vi "读取生成ncx.vi"(8 "error in (no error)":errorcluster caption="错误输入（无错误）", 11 "EPUB输入":refnum<class "EPUB.lvclass">) -> (0 "error out":errorcluster caption="错误输出", 2 "toc.ncx":string, 3 "EPUB输出":refnum<class "EPUB.lvclass">)   [LabVIEW 2016, in "EPUB.lvclass"]
uses:
  EPUB.lvclass
  EPUB.lvclass/EPUB.ctl
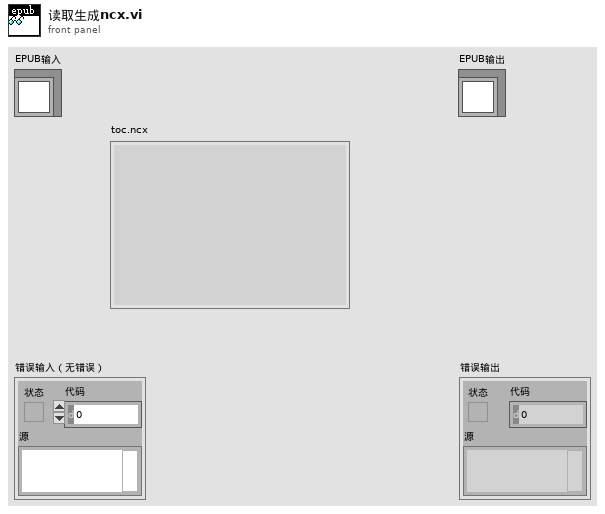
[diagram p1: front panel]
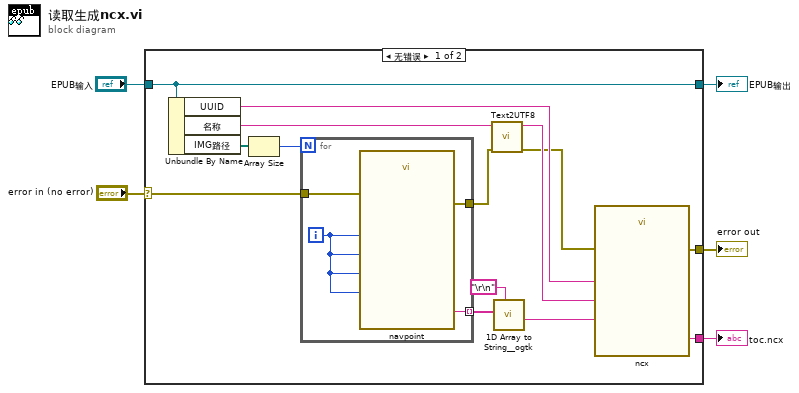
[diagram p0: block diagram]
diagram:
  n1 = case shown="无错误" "error in (no error)" {
    selector: "error in (no error)" -> [w18 w24]
    tunnel: [w10 w24] -> w4
    tunnel: [w19 w25] -> w2
    tunnel: "EPUB输入" -> [w19 w25]
    tunnel: [w11 _] -> w1
    frame No Error {
      n2 = Unbundle By Name(w19) -> ("UUID"=w13:string, "名称"=w14:string, "IMG路径"=w16:path[])
      n3 = Array Size(array=w16) -> (size(s)=w6:i32)
      n4 = for {
        N: w6 -> [_]
        tunnel: w18 -> [w21]
        tunnel: [w23] -> w8
        tunnel: [w22] -> w17 mode=indexing
        i -> [w20]
        n5 = call "navpoint"("idx3"=w20, "idx"=w20, "idx1"=w20, "idx2"=w20, "error in (no error)"=w21) -> ("Result"=w22:string, "error out"=w23:errorcluster)  [unwired: 9 in]
      }
      n6 = call <vilib>:"Text2UTF8.vi"("Error in"=w8, "text"=w14) -> ("Error out"=w7:errorcluster, "utf-8 text"=w9:string)  [unwired: 8 in]
      n7 = call <userlib>:"1D Array to String__ogtk.vi"("delimiter (Tab)"="\r\n", "Array of Strings"=w17) -> ("delimited string"=w12:string)  [unwired: 9 in]
      n8 = call "ncx"("UUID"=w13, "title"=w9, "NAVPOINT"=w12, "error in (no error)"=w7) -> ("Result"=w11:string, "error out"=w10:errorcluster)  [unwired: 10 in]
    }
    frame Error {
    }
  }
  "error out" <- w4
  "EPUB输出" <- w2
  "toc.ncx" <- w1
